vi "程序开始提示.vi"() -> ()   [LabVIEW 2013]
panel:
  out "时间":string
  # "正在进行授权验证，请稍后。。。"
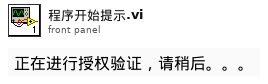
[diagram p1: front panel]
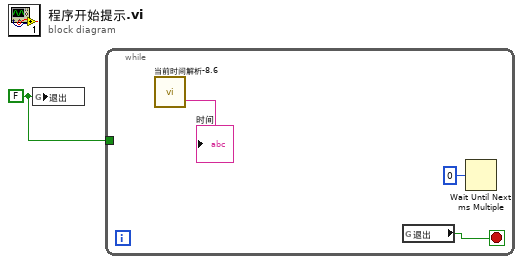
[diagram p0: block diagram]
diagram:
  w1 = FALSE ("退出")
  n1 = global write "EV05全局变量1.vi" "退出"(w1) -> ()
  n2 = while {
    tunnel: w1 -> [_]
    stop <- w4 stop-if-true
    n3 = call "当前时间解析-8.6.vi"() -> ("时间"=→"时间":string)  [unwired: 1 in, 18 out]
    n4 = global read "EV05全局变量1.vi" "退出"() -> (w4:bool)
    n5 = Wait Until Next ms Multiple(millisecond multiple=u32 0 ("毫秒倍数")) -> ()  [unwired: 1 out]
  }
